vi "Test_TerminalVisibility_BooleanFalse_NotVisible.vi"(8 "error in (no error)":errorcluster, 11 "TestCase in":refnum<class "TestTransport.lvclass">) -> (0 "error out":errorcluster, 3 "TestCase out":refnum<class "TestTransport.lvclass">)   [LabVIEW 2017, in "TestTransport.lvclass"]
uses:
  TestTransport.lvclass
  Source/Framework/Transport/TerminalVisibilityBinding/TerminalVisibilityBinding.lvclass
panel:
  out "An I32 Terminal":i32
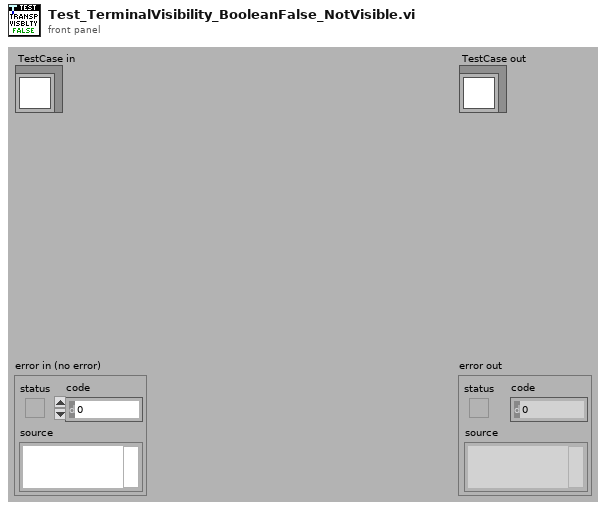
[diagram p1: front panel]
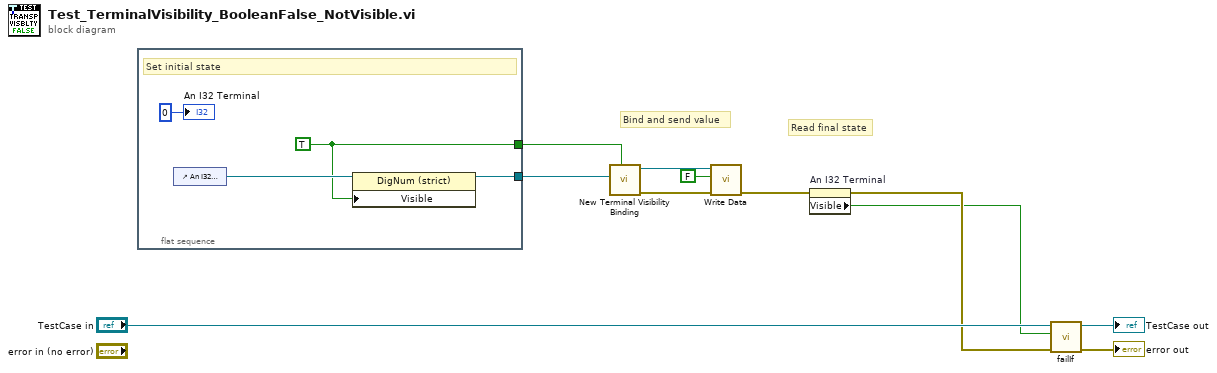
[diagram p0: block diagram]
diagram:
  # "Bind and send value"
  # "Read final state"
  n1 = flat-sequence {
    tunnel: [w13] -> w5
    tunnel: [w12] -> w2
    frame #0 {
      w12 = TRUE ("Visible")
      # "Set initial state"
      n2 = control-ref of="An I32 Terminal"() -> (w14:refnum<vi>)
      n3 = property class="DigNum (strict)"(reference=w14, "Visible"=w12) -> (reference out=w13:refnum<vi>)  [unwired: 1 in, 1 out]
      "An I32 Terminal" <- 0 ("An I32 Terminal")
    }
  }
  n4 = call "New Terminal Visibility Binding.vi"("Initial Visible State (T)"=w2, "Control"=w5) -> ("error out"=w4:errorcluster, "TerminalVisibilityBinding Out"=w8:refnum<class "TerminalVisibilityBinding.lvclass">)  [unwired: 8 in]
  n5 = call-dynamic "Write Data.vi"("error in (no error)"=w4, "Value"=FALSE, "TerminalVisibilityBinding In"=w8) -> ("error out"=w6:errorcluster)  [unwired: 7 in, 1 out]
  n6 = property on="An I32 Terminal" class="DigNum (strict)"(error in=w6) -> (error out=w3:errorcluster, "Visible"=w1:bool)  [unwired: 1 in, 1 out]
  n7 = call-dynamic "failIf.vi"("error in (no error)"=w3, "fail"=w1, "TestCase in"="TestCase in") -> ("error out"=→"error out":errorcluster, "TestCase out"=→"TestCase out":refnum<class "TestTransport.lvclass">)  [unwired: 7 in]
